vi "DAQ_E_mIO_DIO.ProcPeriodic.vi"(0 "i ref in":refnum<vi>, 3 "ms timeout (10000)":i32=10000, 5 "error in (no error)":errorcluster) -> (14 "i ref out":refnum<vi>, 17 "timed out":bool, 19 "error out":errorcluster)   [LabVIEW 2014, in "DAQ_E_mIO_DIO.lvlib"]
doc: "This method serves to periodically do things like reading values from the HW. Methods that should be executed periodically should be called from THIS method. Add code here."
uses:
  DAQ_E_mIO_DIO.lvlib
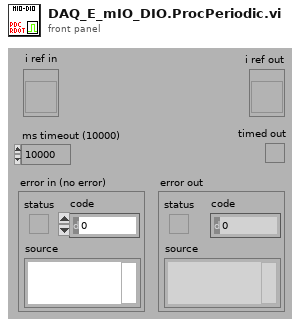
[diagram p1: front panel]
types:
  T1 = typedef "DAQ_E_mIO_DIO.lvlib/DAQ_E_mIO_DIO.i attribute.ctl" = cluster{"DOutChannel":refnum<k21>, "DInChannel":refnum<k21>, "nOfBitsIn":i32, "nOfBitsOut":i32}
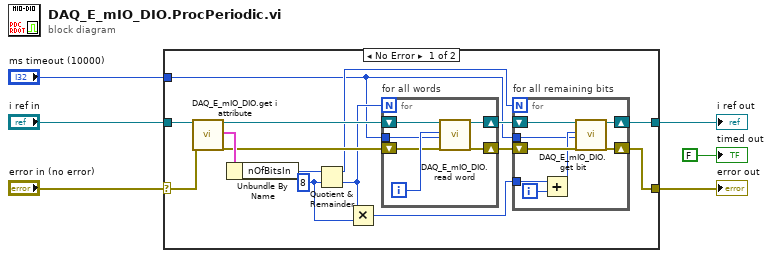
[diagram p0: block diagram]
diagram:
  n1 = case shown="No Error" "error in (no error)" {
    selector: "error in (no error)" -> [w20 w37]
    tunnel: [w12 w37] -> w5
    tunnel: "i ref in" -> [w21 w36]
    tunnel: [w15 w36] -> w3
    tunnel: "ms timeout (10000)" -> [w7 _]
    frame No Error {
      w9 = 8 ("y")
      n2 = call "DAQ_E_mIO_DIO.get i attribute.vi"("i ref in"=w21, "error in (no error)"=w20) -> ("i ref out"=w17:refnum<vi>, "i attribute"=w19:T1, "error out"=w16:errorcluster)  [unwired: 15 in]
      n3 = Unbundle By Name(w19) -> ("nOfBitsIn"=w18:i32)
      n4 = Quotient & Remainder(x=w18, y=w9) -> (x-y*floor(x/y)=w11:i32, floor(x/y)=w10:i32)
      n5 = Multiply(x=w10, y=w9) -> (x*y=w8:i32)
      n6 = for "for all words" {
        N: w10 -> [_]
        tunnel: w7 -> [w33]
        shift-right: [w30] -> w13
        shift-left: w16 -> [w32]
        shift-right: [w31] -> w14
        shift-left: w17 -> [w35]
        i -> [w34]
        n7 = call "DAQ_E_mIO_DIO.read word.vi"("i ref in"=w35, "wordIndex"=w34, "ms timeout (10000)"=w33, "error in (no error)"=w32) -> ("i ref out"=w31:refnum<vi>, "error out"=w30:errorcluster)  [unwired: 12 in, 2 out]
      }
      n8 = for "for all remaining bits" {
        N: w11 -> [_]
        tunnel: w8 -> [w24]
        shift-right: [w26] -> w12
        shift-left: w13 -> [w28]
        shift-right: [w27] -> w15
        shift-left: w14 -> [w29]
        tunnel: w7 -> [w22]
        i -> [w25]
        n9 = Add(x=w24, y=w25) -> (x+y=w23:i32)
        n10 = call "DAQ_E_mIO_DIO.get bit.vi"("i ref in"=w29, "bitIndex"=w23, "ms timeout (10000)"=w22, "error in (no error)"=w28) -> ("i ref out"=w27:refnum<vi>, "error out"=w26:errorcluster)  [unwired: 12 in, 2 out]
      }
    }
    frame Error {
    }
  }
  "error out" <- w5
  "i ref out" <- w3
  "timed out" <- FALSE ("timed out")
